vi "Read Log.vi"(8 "error in (no error)":errorcluster) -> (0 "error out":errorcluster, 3 "log text":string)   [LabVIEW 2017, in "Debug Log.lvlib"]
doc: "Reads the text currently displayed in the debug log.\n\nThis VI executes even if <b>error in</b> has an error."
uses:
  <vilib>/Utility/Debug Log/Debug Log.lvlib
  <vilib>/Utility/Debug Log/Display.vi
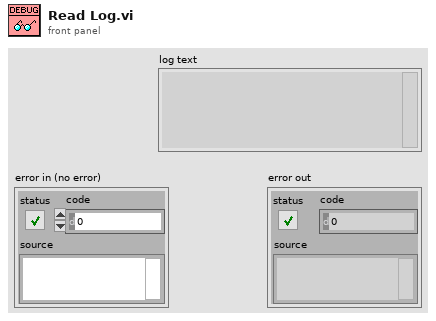
[diagram p1: front panel]
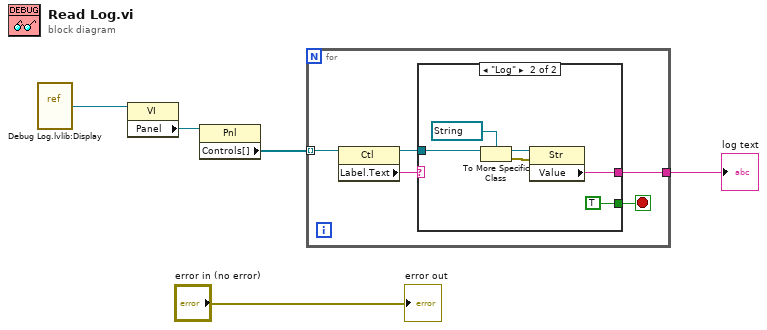
[diagram p0: block diagram]
diagram:
  n1 = vi-ref "Debug Log.lvlib:Display.vi"() -> (w5:refnum<vi>)
  n2 = property class="VI"(reference=w5) -> ("Panel"=w4:refnum<vi>)  [unwired: 1 in, 2 out]
  n3 = property class="Pnl"(reference=w4) -> ("Controls[]"=w3:refnum<vi>[])  [unwired: 1 in, 2 out]
  n4 = for {
    tunnel: w3 -> [w10] mode=indexing
    tunnel: [w7] -> w2
    stop <- w6 stop-if-true
    n5 = property class="Ctl"(reference=w10) -> (reference out=w8:refnum<vi>, "Label.Text"=w9:string)  [unwired: 1 in, 1 out]
    n6 = case shown="\"Log\"" w9 {
      tunnel: w8 -> [_ w16]
      tunnel: [_ w12] -> w7
      tunnel: [_ TRUE] -> w6
      frame Default {
      }
      frame "Log" {
        n7 = To More Specific Class(target class=refnum<vi> refnum ("Log"), reference=w16) -> (specific class reference=w14:refnum<vi>, error out=w13:errorcluster)  [unwired: 1 in]
        n8 = property class="Str"(reference=w14, error in=w13) -> ("Value"=w12:string)  [unwired: 2 out]
      }
    }
  }
  "log text" <- w2
  "error out" <- "error in (no error)"
